vi "Read Objects.vi"(8 "error in":errorcluster, 9 "count (-1: all)":i32=-1, 11 "ByteBuffer in":refnum<data-value>) -> (0 "error out":errorcluster, 2 "elements":refnum<class>[](array[class]), 3 "ByteBuffer":refnum<data-value>)   [LabVIEW 2013, in "CircularBuffer.lvlib" / "ObjectBuffer.lvclass"]
doc: "This VI returns data from the ring buffer starting from the oldest data and ending with the newest.\n\nThe data is duplicated at the output so this VI allocates new place in the memory for the output."
uses:
  ObjectBuffer.lvclass
  VariantBuffer/VariantBuffer.lvclass
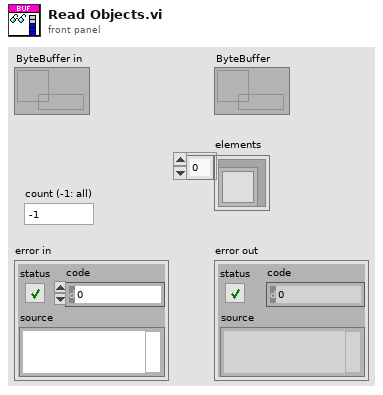
[diagram p1: front panel]
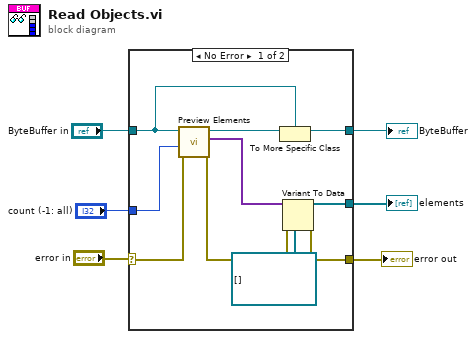
[diagram p0: block diagram]
diagram:
  n1 = case shown="No Error" "error in" {
    selector: "error in" -> [w14 w17]
    tunnel: "ByteBuffer in" -> [w8 w18]
    tunnel: [w9 w18] -> w1
    tunnel: [w10 w17] -> w3
    tunnel: [w12 _] -> w2
    tunnel: "count (-1: all)" -> [w15 _]
    frame No Error {
      n2 = call "Preview Elements.vi"("error in"=w14, "count (-1: all)"=w15, "ByteBuffer in"=w8) -> ("error out"=w11:errorcluster, "elements"=w13:variant[], "ByteBuffer"=w16:refnum<data-value>)  [unwired: 6 in]
      n3 = To More Specific Class(target class=w8, reference=w16) -> (specific class reference=w9:refnum<data-value>)  [unwired: 1 in, 1 out]
      n4 = Variant To Data(error in=w11, type=refnum<class>[] [] ("elements"), Variant=w13) -> (data=w12:refnum<class>[], error out=w10:errorcluster)
    }
    frame Error {
    }
  }
  "error out" <- w3
  "ByteBuffer" <- w1
  "elements" <- w2
